vi "izamax - Max Element Index (CDB).vi"(7 "xInc":i32=1, 11 "x":cdb[](array[numeric])) -> (0 "error":i32, 3 "izamax":i32)   [LabVIEW 2017, in "NI_AALBLAS.lvlib"]
doc: "For real vectors, returns the index of the element that has the maximum absolute value. For complex vectors, the VI returns the index of the element that has the maximum sum of absolute real and imaginary parts."
uses:
  <vilib>/Analysis/NI_AALBLAS.lvlib
  <vilib>/Analysis/BLAS.llb/Fucntion.ctl
  <vilib>/Analysis/BLAS.llb/BLAS1 Utility(CDB).vi
panel:
  # "izamax=the index of max(|Re(x)|+|Im(x)|)"
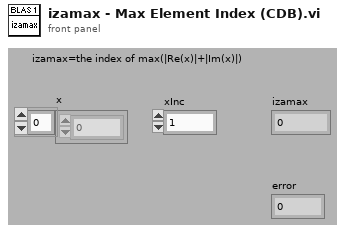
[diagram p1: front panel]
types:
  T1 = typedef "NI_AALBLAS.lvlib/Fucntion.ctl" = u16
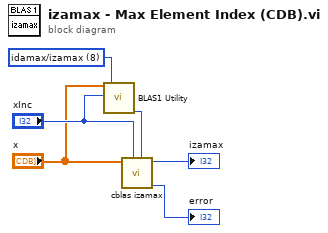
[diagram p0: block diagram]
diagram:
  w1 = T1 8 items=["ddot/zdotu/zdotc", "daxpy/zaxpy", "dnrm2/dznrm2", "dasum/dzasum", "dcopy/zcopy", "dswap/zswap", "drotm", "drot/zdrot", "idamax/izamax", "idamin/izamin", "dgemv/zgemv", "dsymv/zhemv", "dtrmv/ztrmv", "dsyr/zher", "dsyr2/zher2", "dger/zgeru/zgerc", "dtrsv/ztrsv", "dgemm/zgemm", "dsymm/zsymm/zhemm", "dtrmm/ztrmm", "dsyrk/zsyrk/zherk", "dsyr2k/zsyr2k/zher2k", "dtrsm/ztrsm"] ("function")
  n1 = call-poly <vilib>:"BLAS1 Utility.vi"("x"="x", "xInc"="xInc", "function"=w1) -> ("n"=w2:i32)  [unwired: 2 in, 14 out]
  n2 = call <vilib>:"cblas izamax.vi"("n"=w2, "incx"="xInc", "x"="x") -> ("error"=→"error":i32, "izamax"=→"izamax":i32)  [unwired: 7 out]
